vi "finishUp.vi"(8 "error in (no error)":errorcluster, 11 "RampAction in":refnum<class "RampAction.lvclass">) -> (0 "error out":errorcluster, 3 "RampAction out":refnum<class "RampAction.lvclass">)   [LabVIEW 2009, in "Views.lvlib" / "ScriptEditor.lvlib" / "RampAction.lvclass"]
uses:
  RampAction.lvclass
  RampAction.lvclass/RampAction.ctl
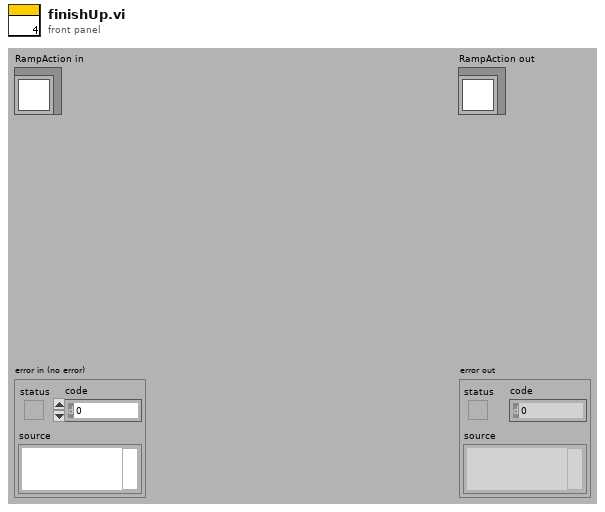
[diagram p1: front panel]
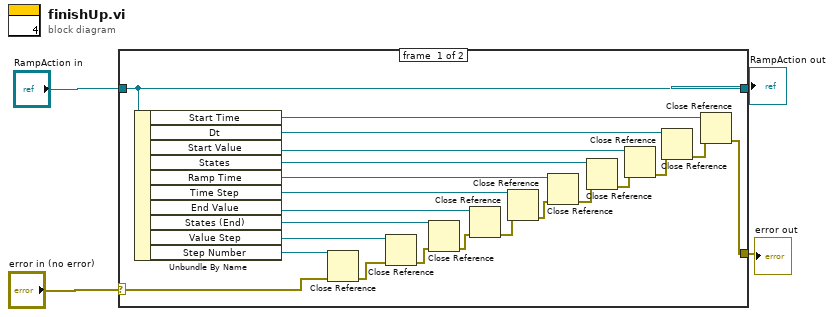
[diagram p0: block diagram]
diagram:
  n1 = case shown="No Error" "error in (no error)" {
    selector: "error in (no error)" -> [w6 w27]
    tunnel: "RampAction in" -> [w26 w28]
    tunnel: [w8 w27] -> w2
    tunnel: [w26 w28] -> w1
    frame #0 {
      n2 = Unbundle By Name(w26) -> ("Start Time"=w17:refnum<vi>, "Dt"=w18:refnum<vi>, "Start Value"=w19:refnum<vi>, "States"=w20:refnum<vi>, "Ramp Time"=w21:refnum<vi>, "Time Step"=w22:refnum<vi>, "End Value"=w23:refnum<vi>, "States (End)"=w24:refnum<vi>, "Value Step"=w25:refnum<vi>, "Step Number"=w7:refnum<vi>)
      n3 = Close Reference(reference=w7, error in (no error)=w6) -> (error out=w5:errorcluster)
      n4 = Close Reference(reference=w25, error in (no error)=w5) -> (error out=w9:errorcluster)
      n5 = Close Reference(reference=w24, error in (no error)=w9) -> (error out=w10:errorcluster)
      n6 = Close Reference(reference=w23, error in (no error)=w10) -> (error out=w11:errorcluster)
      n7 = Close Reference(reference=w22, error in (no error)=w11) -> (error out=w12:errorcluster)
      n8 = Close Reference(reference=w21, error in (no error)=w12) -> (error out=w13:errorcluster)
      n9 = Close Reference(reference=w20, error in (no error)=w13) -> (error out=w14:errorcluster)
      n10 = Close Reference(reference=w19, error in (no error)=w14) -> (error out=w15:errorcluster)
      n11 = Close Reference(reference=w18, error in (no error)=w15) -> (error out=w16:errorcluster)
      n12 = Close Reference(reference=w17, error in (no error)=w16) -> (error out=w8:errorcluster)
    }
    frame #1 {
    }
  }
  "error out" <- w2
  "RampAction out" <- w1
